vi "formantDAQ.vi"() -> ()   [LabVIEW 2012]
uses:
  <vilib>/silver_ctls/ArrayMatrixCluster/Real Matrix NI_Silver.ctl
  <vilib>/Analysis/3filter.llb/FIR Filter (DBL).vi
  <vilib>/Analysis/baseanly.llb/Mean (DBL).vi
  <vilib>/Utility/file.llb/Read From Spreadsheet File (DBL).vi
  <vilib>/Analysis/2dsp.llb/Real FFT.vi
  <vilib>/Analysis/2dsp.llb/1D DCT.vi
  <vilib>/Utility/file.llb/Write To Spreadsheet File (DBL).vi
  <vilib>/Analysis/4window.llb/Hamming Window (DBL).vi
  <vilib>/Analysis/NI_AALBase.lvlib
  <vilib>/Analysis/NI_AALPro.lvlib
  <vilib>/Analysis/NI_AAL_SigProc.lvlib
panel:
  out "min wartość":dbl
  out "Min. indeks":i32
  out "wynik":dbl[](array[numeric])
  out "Dane rozpoznawane":T1
  out "Dane zapisane":T1
  in  "pomiar":bool=TRUE
  in  "licz":bool
  out "Mowa wejściowa":waveform(dbl)[](graph)
  out "Częstotliwości środka":dbl[](array[numeric])
  out "Wypowiedź":dbl[](graph)
  out "min index":dbl
  out "max index":dbl
  out "\"Uproszczona\" energia":dbl[](graph)
  out "Długość":dbl
  out "Suma":dbl
  out "size(s)":i32
  out "diagram energii":dbl[](graph)
  out "Energia progowa":dbl
  out "number of rows":i32
  out "number of columns":i32
  out "Tablica ramek":dbl[](graph)
  out "Przekroczenie progu":bool
  out "Ramki":dbl[][](array[numeric])
  out "Energia sygnału":dbl
  in  "stop":bool
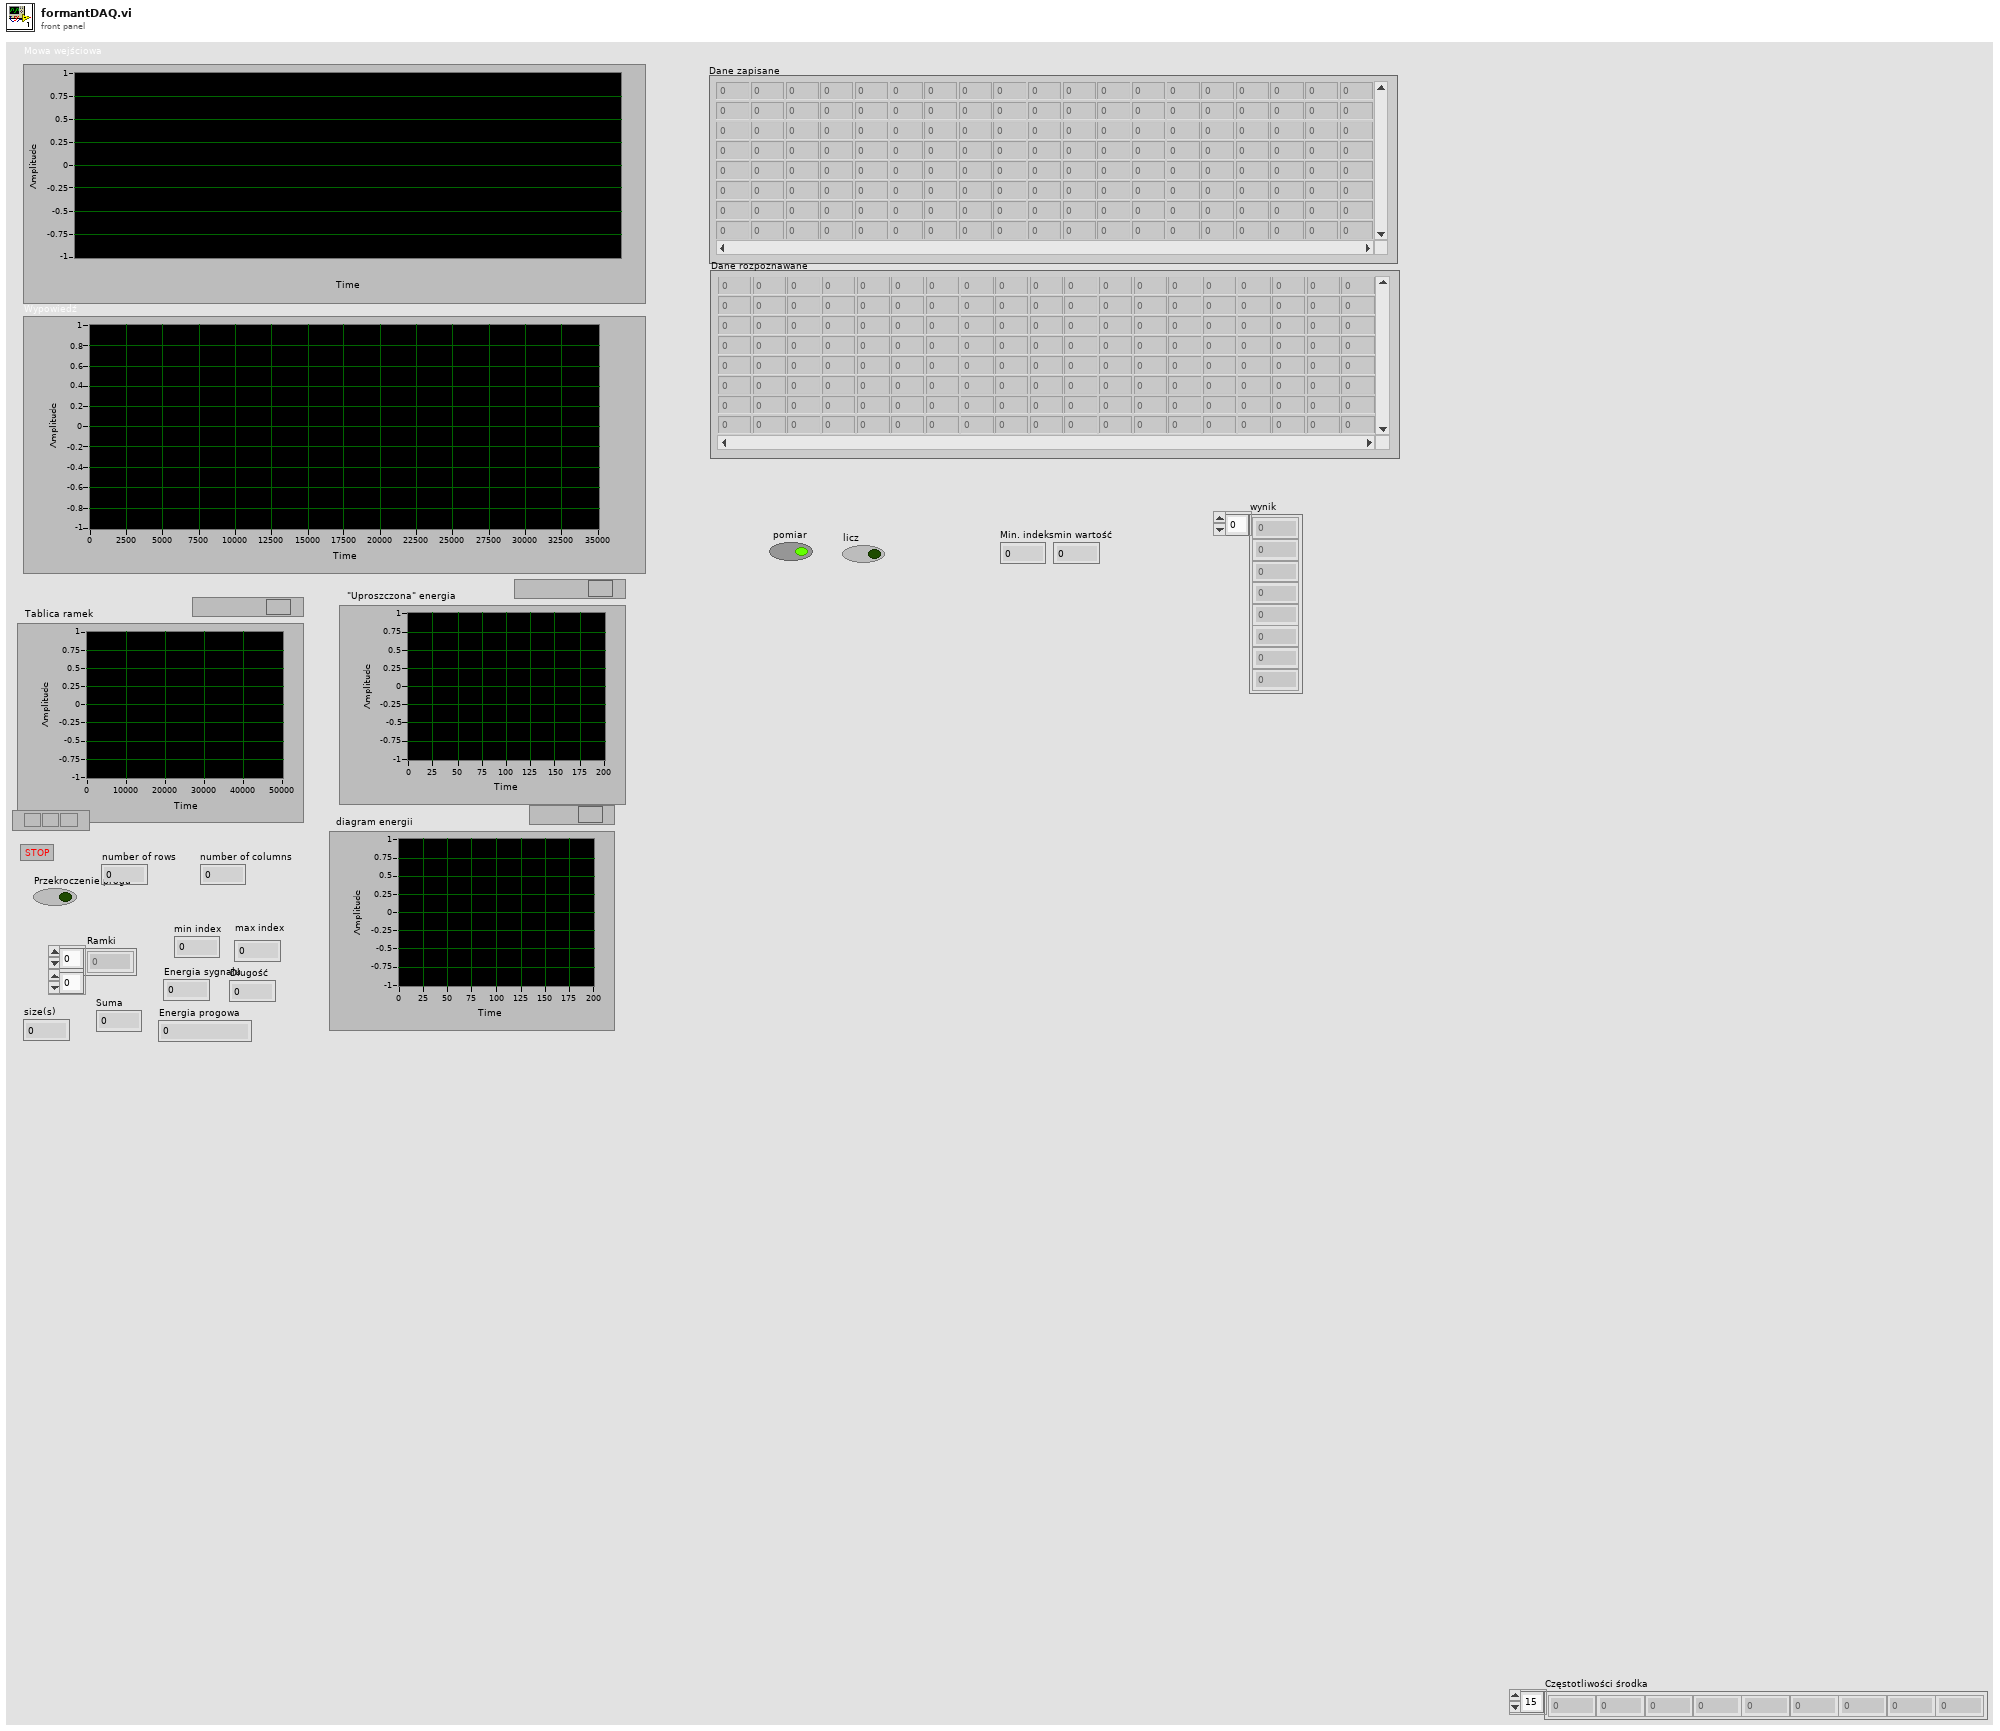
[diagram p1: front panel]
types:
  T1 = typedef "Real Matrix NI_Silver.ctl" = dbl[][]
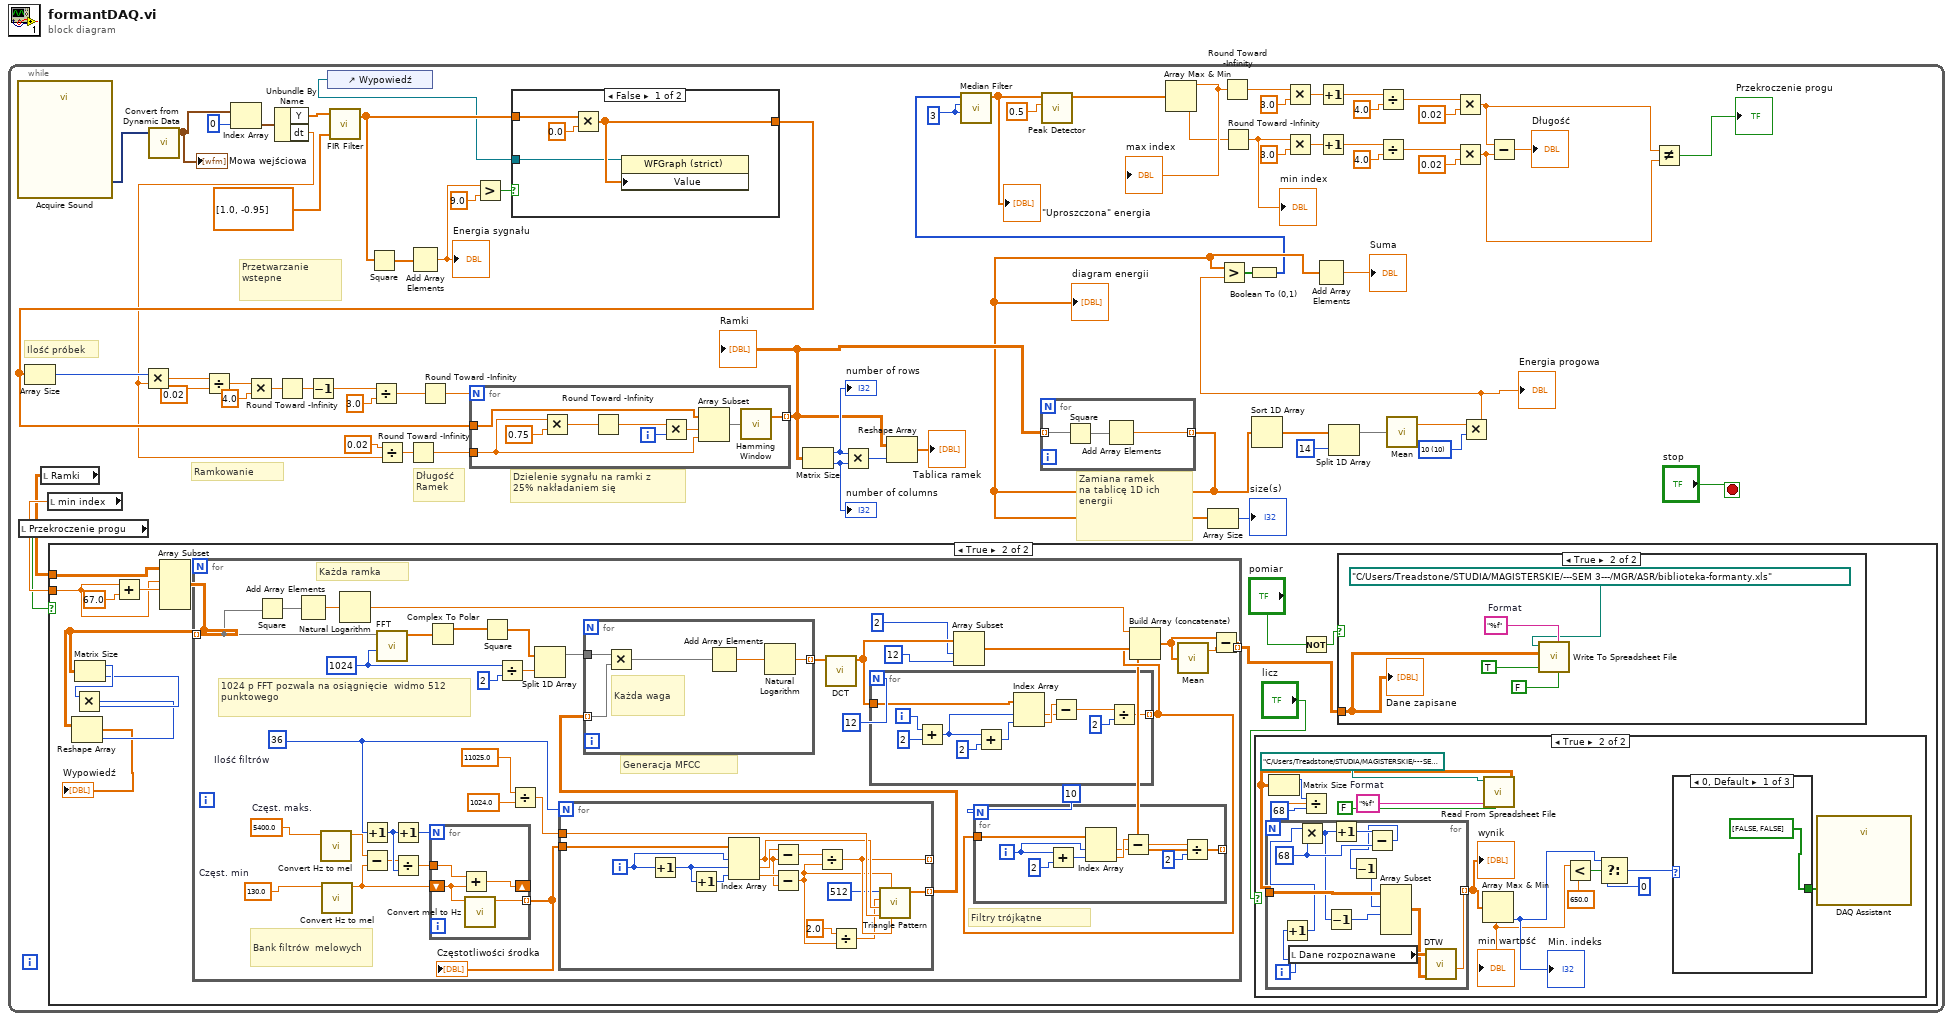
[diagram p0: block diagram]
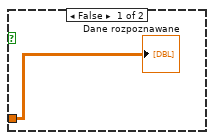
[diagram p3: hidden frame]
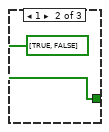
[diagram p5: hidden frame]
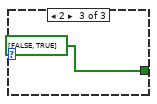
[diagram p6: hidden frame]
diagram:
  n1 = while {
    stop <- "stop" stop-if-true
    w16 = 3 ("right rank")
    w40 = u16 10 items=["5"=5, "6"=6, "7"=7, "9"=9, "10"=10]
    # "Ramkowanie"
    # "Przetwarzanie \nwstepne"
    # "Zamiana ramek  \nna tablicę 1D ich \nenergii"
    # "Dzielenie sygnału na ramki z \n25% nakładaniem się"
    # "Długość\nRamek"
    # "Ilość próbek"
    n2 = call "Acquire Sound"() -> ("Data"=w72:dynamicdata)  [unwired: 18 in, 1 out]
    n3 = local read "Przekroczenie progu"() -> (w2:bool)
    n4 = local read "Ramki"() -> (w3:dbl[][])
    n5 = local read "min index"() -> (w4:dbl)
    n6 = case shown="True" w2 {
      tunnel: w4 -> [_ w79]
      tunnel: w3 -> [_ w80]
      frame False {
      }
      frame True {
        n7 = Add(x=w79, y=67.0 ("x")) -> (x+y=w84:dbl)
        n8 = Array Subset(array=w80, index (row)=w79, length (row)=w84) -> (w77:dbl[][])  [unwired: 2 in]
        n9 = Matrix Size(0:w77) -> (1:w83:i32, 2:w82:i32)
        n10 = Multiply(x=w83, y=w82) -> (x*y=w81:i32)
        n11 = Reshape Array(w77, w81) -> (→"Wypowiedź":dbl[])
        n12 = for {
          tunnel: w77 -> [w150] mode=indexing
          tunnel: [w125] -> w76 mode=indexing
          w154 = 1024 ("FFT size")
          w129 = 36  # Ilość filtrów
          w127 = 5400.0  # Częst. maks.
          w128 = 130.0  # Częst. min
          # "Filtry trójkątne"
          # "Bank filtrów  melowych"
          # "Każda ramka"
          # "Generacja MFCC"
          # "1024 p FFT pozwala na osiągnięcie  widmo 512  punktowego"
          n13 = Square(x=w150) -> (x^2=w149:dbl[])
          n14 = Add Array Elements(numeric array=w149) -> (sum=w148:dbl)
          n15 = call "Convert Hz to mel.vi"("Hz"=w127) -> ("mel"=w131:dbl)  [unwired: 10 in]
          n16 = call "Convert Hz to mel.vi"("Hz"=w128) -> ("mel"=w134:dbl)  [unwired: 10 in]
          n17 = Natural Logarithm(1:w148) -> (0:w144:dbl)
          n18 = Increment(x=w129) -> (x+1=w135:i32)
          n19 = Subtract(x=w131, y=w134) -> (x-y=w132:dbl)
          n20 = call-poly <vilib>:"FFT.vi"("FFT size"=w154, "X"=w150) -> ("FFT {X}"=w156:cdb[])  [unwired: 8 in, 1 out]
          n21 = Increment(x=w135) -> (x+1=w130:i32)
          n22 = Divide(x=w132, y=w135) -> (x/y=w133:dbl)
          n23 = Complex To Polar(r * e^(i*theta)=w156) -> (r=w155:dbl[])  [unwired: 1 out]
          n24 = for {
            N: w130 -> [_]
            tunnel: w133 -> [w175]
            tunnel: [w177] -> w139 mode=indexing
            shift-right: [w174] -> _
            shift-left: w134 -> [w176]
            n25 = Add(x=w175, y=w176) -> (x+y=w174:dbl)
            n26 = call "Convert mel to Hz.vi"("mel"=w176) -> ("Hz"=w177:dbl)  [unwired: 10 in]
          }
          "Częstotliwości środka" <- w139
          n27 = Square(x=w155) -> (x^2=w151:dbl[])
          n28 = Divide(x=w154, y=2 ("FFT size")) -> (x/y=w152:dbl)
          n29 = Divide(x=11025.0, y=1024.0) -> (x/y=w138:dbl)
          n30 = Split 1D Array(array=w151, index=w152) -> (first subarray=w158:dbl[])  [unwired: 1 out]
          n31 = for {
            N: w129 -> [_]
            tunnel: [w170] -> w126 mode=indexing
            tunnel: w139 -> [w169]
            tunnel: w138 -> [w168]
            tunnel: [w163] -> _ mode=indexing
            i -> [w173]
            n32 = Increment(x=w173) -> (x+1=w172:i32)
            n33 = Increment(x=w172) -> (x+1=w171:i32)
            n34 = Index Array(array=w169, index #1=w173, index #2=w172, index #3=w171) -> (element #1=w165:dbl, element #2=w166:dbl, element #3=w167:dbl)
            n35 = Subtract(x=w166, y=w165) -> (x-y=w164:dbl)
            n36 = Subtract(x=w167, y=w165) -> (x-y=w162:dbl)
            n37 = Divide(x=w164, y=w162) -> (x/y=w163:dbl)
            n38 = Divide(x=2.0, y=w162) -> (x/y=w160:dbl)
            n39 = call <vilib>:"Triangle Pattern.vi"("asymmetry"=w163, "width (s)"=w162, "delta t (s)"=w168, "delay (s)"=w165, "amplitude"=w160, "samples"=512) -> ("Triangle Pattern"=w170:dbl[])  [unwired: 4 in, 1 out]
          }
          n40 = for {
            tunnel: w126 -> [w201] mode=indexing
            tunnel: [w199] -> w157 mode=indexing
            tunnel: w158 -> [w198]
            # "Każda waga"
            n41 = Multiply(x=w198, y=w201) -> (x*y=w202:dbl[])
            n42 = Add Array Elements(numeric array=w202) -> (sum=w200:dbl)
            n43 = Natural Logarithm(1:w200) -> (0:w199:dbl)
          }
          n44 = call-poly <vilib>:"DCT.vi"("X"=w157) -> ("DCT {X}"=w146:dbl[])  [unwired: 9 in, 1 out]
          n45 = for {
            N: 12 -> [_]
            tunnel: w146 -> [w197]
            tunnel: [w190] -> w123 mode=indexing
            i -> [w195]
            n46 = Add(x=w195, y=2) -> (x+y=w187:i32)
            n47 = Add(x=w187, y=2) -> (x+y=w188:i32)
            n48 = Index Array(array=w197, index #1=w187, index #2=w188) -> (element #1=w193:dbl, element #2=w194:dbl)
            n49 = Subtract(x=w194, y=w193) -> (x-y=w192:dbl)
            n50 = Divide(x=w192, y=2) -> (x/y=w190:dbl)
          }
          n51 = Array Subset(array=w146, index=2, length=12 ("index")) -> (w143:dbl[])
          n52 = for {
            N: 10 -> [_]
            tunnel: w123 -> [w186]
            tunnel: [w180] -> w122 mode=indexing
            i -> [w179]
            n53 = Add(x=w179, y=2) -> (x+y=w178:i32)
            n54 = Index Array(array=w186, index #1=w179, index #2=w178) -> (element #1=w183:dbl, element #2=w184:dbl)
            n55 = Subtract(x=w184, y=w183) -> (x-y=w182:dbl)
            n56 = Divide(x=w182, y=2) -> (x/y=w180:dbl)
          }
          n57 = Build Array (concatenate)(w144, w143, w123, w122) -> (w141:dbl[])
          n58 = call-poly <vilib>:"Mean.vi"("X"=w141) -> ("mean"=w142:dbl)  [unwired: 1 out]
          n59 = Subtract(x=w141, y=w142) -> (x-y=w125:dbl[])
        }
        n60 = case shown="True" "licz" {
          frame False {
          }
          frame True {
            w105 = "%f"  # Format
            n61 = call-poly <vilib>:"Read From Spreadsheet File.vi"("transpose (no:F)"=FALSE, "format (%.3f)"=w105, "file path (dialog if empty)"=path "C:/Users/Treadstone/STUDIA/MAGISTERSKIE/---SEM 3---/MGR/ASR/biblioteka-formanty.xls") -> ("all rows"=w101:dbl[][])  [unwired: 4 in, 4 out]
            n62 = Matrix Size(0:w101) -> (1:w103:i32)  [unwired: 1 out]
            n63 = Divide(x=w103, y=68) -> (x/y=w100:dbl)
            n64 = for {
              N: w100 -> [_]
              tunnel: w101 -> [w118]
              tunnel: [w115] -> w99 mode=indexing
              i -> [w113]
              w120 = 68
              n65 = Increment(x=w113) -> (x+1=w112:i32)
              n66 = local read "Dane rozpoznawane"() -> (w117:T1)
              n67 = Multiply(x=w112, y=w120) -> (x*y=w114:i32)
              n68 = Decrement(x=w114) -> (x-1=w110:i32)
              n69 = Increment(x=w114) -> (x+1=w121:i32)
              n70 = Subtract(x=w121, y=w120) -> (x-y=w119:i32)
              n71 = Decrement(x=w119) -> (x-1=w111:i32)
              n72 = Array Subset(array=w118, index (row)=w111, length (row)=w110) -> (w116:dbl[][])  [unwired: 2 in]
              n73 = call "DTW.vi"("Reference Sequence"=w116, "Test Sequence"=w117) -> ("Cost"=w115:dbl)  [unwired: 9 in]
            }
            "wynik" <- w99
            n74 = Array Max & Min(array=w99) -> (min value=w92:dbl, min index (indices)=w93:i32)  [unwired: 2 out]
            "Min. indeks" <- w93
            "min wartość" <- w92
            n75 = Less?(x=w92, y=650.0) -> (x < y?=w97:bool)
            n76 = Select(t=w93, s=w97, f=0) -> (s? t:f=w94:i32)
            n77 = case shown="0, Default" w94 {
              tunnel: [bool[] [FALSE, FALSE] ("data") bool[] [TRUE, FALSE] ("data") bool[] [FALSE, TRUE] ("data")] -> w98
              frame 0, Default {
              }
              frame 1 {
              }
              frame 2 {
              }
            }
            n78 = call "DAQ Assistant"("data"=w98) -> ()  [unwired: 17 in, 2 out]
          }
        }
        n79 = Not(x="pomiar") -> (.not. x?=w73:bool)
        n80 = case shown="True" w73 {
          tunnel: w76 -> [w86 w88]
          frame False {
            "Dane rozpoznawane" <- w86
          }
          frame True {
            w91 = "%f"  # Format
            n81 = call-poly <vilib>:"Write To Spreadsheet File.vi"("transpose? (no:F)"=FALSE, "format (%.3f)"=w91, "append to file? (new file:F)"=TRUE, "2D data"=w88, "file path (dialog if empty)"=path "C:/Users/Treadstone/STUDIA/MAGISTERSKIE/---SEM 3---/MGR/ASR/biblioteka-formanty.xls") -> ()  [unwired: 3 in, 1 out]
            "Dane zapisane" <- w88
          }
        }
      }
    }
    n82 = call "Convert from Dynamic Data"("Dynamic Data Type"=w72) -> ("Array of Waveform"=w1:waveform(dbl)[])  [unwired: 3 in]
    "Mowa wejściowa" <- w1
    n83 = Index Array(array=w1, index=0) -> (element=w62:waveform(dbl))
    n84 = Unbundle By Name(w62) -> ("Y"=w61:dbl[], "dt"=w41:dbl)
    n85 = control-ref of="Wypowiedź"() -> (w5:refnum<vi>)
    n86 = call-poly <vilib>:"FIR Filter.vi"("FIR Coefficients"=dbl[] [1.0, -0.95], "X"=w61) -> ("Filtered X"=w70:dbl[])  [unwired: 2 in, 1 out]
    n87 = Square(x=w70) -> (x^2=w66:dbl[])
    n88 = Divide(x=0.02, y=w41) -> (x/y=w47:dbl)
    n89 = Round Toward -Infinity(1:w47) -> (0:w48:dbl)
    n90 = Add Array Elements(numeric array=w66) -> (sum=w68:dbl)
    "Energia sygnału" <- w68
    n91 = Greater?(x=w68, y=9.0) -> (0:w69:bool)
    n92 = case shown="False" w69 {
      tunnel: w70 -> [w217 w219]
      tunnel: [w216 w219] -> w42
      tunnel: w5 -> [w215 _]
      frame False {
        n93 = Multiply(x=w217, y=0.0) -> (x*y=w216:dbl[])
        n94 = property class="WFGraph (strict)"(reference=w215, "Value"=w216) -> ()  [unwired: 1 in, 2 out]
      }
      frame True {
      }
    }
    n95 = Array Size(array=w42) -> (size(s)=w60:i32)
    n96 = Multiply(x=w60, y=w41) -> (x*y=w58:dbl)
    n97 = Divide(x=w58, y=0.02) -> (x/y=w54:dbl)
    n98 = Multiply(x=w54, y=4.0) -> (x*y=w53:dbl)
    n99 = Round Toward -Infinity(1:w53) -> (0:w56:dbl)
    n100 = Decrement(x=w56) -> (x-1=w51:dbl)
    n101 = Divide(x=w51, y=3.0) -> (x/y=w50:dbl)
    n102 = Round Toward -Infinity(1:w50) -> (0:w49:dbl)
    n103 = for {
      N: w49 -> [_]
      tunnel: w42 -> [w214]
      tunnel: w48 -> [w211]
      tunnel: [w206] -> w32 mode=indexing
      i -> [w213]
      n104 = Multiply(x=w211, y=0.75 ("x")) -> (x*y=w209:dbl)
      n105 = Round Toward -Infinity(1:w209) -> (0:w208:dbl)
      n106 = Multiply(x=w208, y=w213) -> (x*y=w210:dbl)
      n107 = Array Subset(array=w214, index=w210, length=w211) -> (w207:dbl[])
      n108 = call-poly <vilib>:"Hamming Window.vi"("X"=w207) -> ("Windowed X"=w206:dbl[])  [unwired: 1 out]
    }
    "Ramki" <- w32
    n109 = Matrix Size(0:w32) -> (1:w46:i32, 2:w45:i32)
    "number of columns" <- w45
    "number of rows" <- w46
    n110 = Multiply(x=w46, y=w45) -> (x*y=w44:i32)
    n111 = Reshape Array(w32, w44) -> (→"Tablica ramek":dbl[])
    n112 = for {
      tunnel: w32 -> [w205] mode=indexing
      tunnel: [w203] -> w9 mode=indexing
      n113 = Square(x=w205) -> (x^2=w204:dbl[])
      n114 = Add Array Elements(numeric array=w204) -> (sum=w203:dbl)
    }
    "diagram energii" <- w9
    n115 = Array Size(array=w9) -> (size(s)=→"size(s)":i32)
    n116 = Sort 1D Array(array=w9) -> (sorted array=w36:dbl[])
    n117 = Add Array Elements(numeric array=w9) -> (sum=→"Suma":dbl)
    n118 = Split 1D Array(array=w36, index=14) -> (first subarray=w34:dbl[])  [unwired: 1 out]
    n119 = call-poly <vilib>:"Mean.vi"("X"=w34) -> ("mean"=w33:dbl)  [unwired: 1 out]
    n120 = Multiply(x=w33, y=w40) -> (x*y=w39:dbl)
    "Energia progowa" <- w39
    n121 = Greater?(x=w9, y=w39) -> (0:w38:bool[])
    n122 = Boolean To (0,1)(Boolean=w38) -> (0, 1=w6:i16[])
    n123 = call <vilib>:"Median Filter.vi"("right rank"=w16, "left rank"=w16, "X"=w6) -> ("Filtered X"=w13:dbl[])  [unwired: 7 in, 1 out]
    "\"Uproszczona\" energia" <- w13
    n124 = call <vilib>:"Peak Detector.vi"("threshold"=0.5, "X"=w13) -> ("Locations"=w15:dbl[])  [unwired: 5 in, 4 out]
    n125 = Array Max & Min(array=w15) -> (max value=w17:dbl, min value=w12:dbl)  [unwired: 2 out]
    "max index" <- w17
    n126 = Round Toward -Infinity(1:w17) -> (0:w30:dbl)
    n127 = Round Toward -Infinity(1:w12) -> (0:w11:dbl)
    "min index" <- w11
    n128 = Multiply(x=w30, y=3.0) -> (x*y=w19:dbl)
    n129 = Multiply(x=w11, y=3.0) -> (x*y=w28:dbl)
    n130 = Increment(x=w19) -> (x+1=w20:dbl)
    n131 = Increment(x=w28) -> (x+1=w27:dbl)
    n132 = Divide(x=w20, y=4.0) -> (x/y=w22:dbl)
    n133 = Divide(x=w27, y=4.0) -> (x/y=w25:dbl)
    n134 = Multiply(x=w22, y=0.02) -> (x*y=w8:dbl)
    n135 = Multiply(x=w25, y=0.02) -> (x*y=w7:dbl)
    n136 = Subtract(x=w8, y=w7) -> (x-y=→"Długość":dbl)
    n137 = Not Equal?(x=w8, y=w7) -> (x != y?=→"Przekroczenie progu":bool)
  }
